vi "test Verify Class Roster as JSON.vi"(8 "error in":errorcluster, 11 "Testing Approval Tests in":refnum<class "VITester Extension Tests.lvclass">) -> (0 "error out":errorcluster, 3 "Testing Approval Tests out":refnum<class "VITester Extension Tests.lvclass">)   [LabVIEW 2026, in "VITester Extension Tests.lvclass"]
uses:
  VITester Extension Tests.lvclass
  C:/Program Files/National Instruments/LabVIEW 2026/vi.lib/Addons/_JKI Toolkits/VI Tester/TestCase.llb/TestCase.lvclass
  Source/Extensions/VITester.Extension/VITester.Extension.lvlib
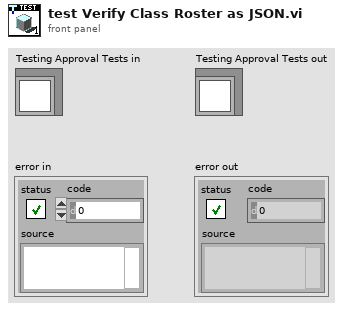
[diagram p1: front panel]
types:
  T1 = cluster{"Subject":string, "Teacher":cluster{"First Name":string, "Last Name":string}, "Assignments":cluster{"Description":string, "Grades":map{cluster{"First Name":string, "Last Name":string}, i32}}[], "Roster":cluster{"First Name":string, "Last Name":string}[]}
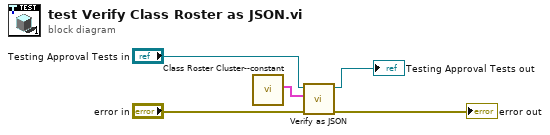
[diagram p0: block diagram]
diagram:
  n1 = call "Class Roster Cluster--constant.vi"() -> ("Class Roster"=w1:T1)  [unwired: 11 in]
  n2 = call "Verify as JSON.vi"("error in"="error in", "Anything"=w1, "TestCase in"="Testing Approval Tests in") -> ("error out"=→"error out":errorcluster, "TestCase out"=→"Testing Approval Tests out":refnum<class "VITester Extension Tests.lvclass">)  [unwired: 7 in]
